vi "FIR Windowed Filter Design - DFD.vi"() -> ()   [LabVIEW 2023]
doc: "Demonstrates how to design an FIR windowed filter using VIs in the LabVIEW Digital Filter Design Toolkit. \n\nAs you change the Filter Type, experiment with the parameters for that filter type and observe their effect on the magnitude and phase responses."
uses:
  <vilib>/addons/Digital Filter Design/_Objects.llb/DFD Phase Setting.ctl
  <vilib>/addons/Digital Filter Design/Analysis.llb/DFD Plot Freq Response (Linear-Spaced).vi
  <vilib>/addons/Digital Filter Design/NI_DigFilterLicensed.lvlib
panel:
  out "?":string="dB"
  in  "window":i32(ring)=1 items=["None", "Hanning", "Hamming", "Triangular", "Blackman", "Exact Blackman", "Blackman-Harris", "Kaiser-Bessel", "Flat Top"]
  in  "high cutoff freq: fh":dbl=350.0 format="%0.2f"
  in  "low cutoff freq: fl":dbl=150.0 format="%0.2f"
  in  "sampling frequency: fs":dbl=1000.0 format="%0.2f"
  in  "Display":bool=TRUE
  in  "stop":bool
  in  "Filter Type":T1(ring)=enum."Bandpass"
  in  "taps":i32=33
  out "Phase Response":cluster{"f0":dbl, "df":dbl, "values":dbl[]}[](graph)
  out "Magnitude Response":cluster{"f0":dbl, "df":dbl, "values":dbl[]}[](graph)
  # "Select Help»Show Context Help and move the cursor over the VI icon for more information."
  # "Hz"
  # "radians"
  # "Hz"
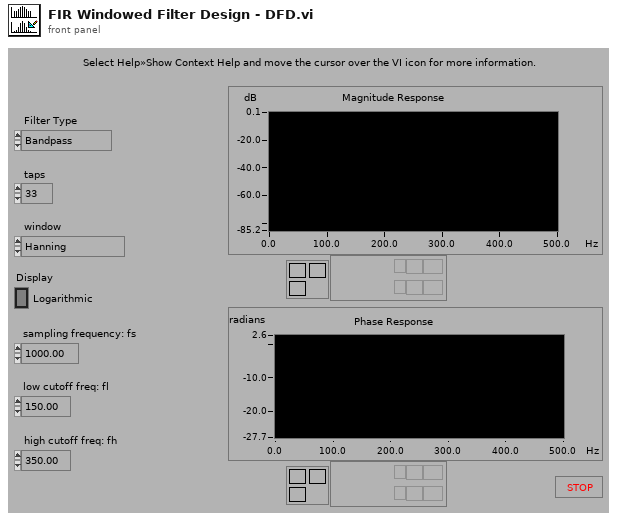
[diagram p1: front panel]
types:
  T1 = enum16{"Lowpass", "Highpass", "Bandpass", "Bandstop"}
  T2 = typedef "NI_DigFilterLicensed.lvlib/DFD Phase Setting.ctl" = cluster{"unwrap? (F)":bool, "degree? (F)":bool}
  T3 = typedef "NI_DigFilterLicensed.lvlib/DFD Filter Obj.ctl" = cluster{"mSRate_Fs":dbl, "mSRate_Version":string, "mSRate_Comments":string, "mSRate_OrgCoef":T4, "mSRate_CurCoef":T4, "mSRate_Quantized?":bool, "mSRate_QCoef":T4, "mSRate_QSettings":T6[], "mSRate_Order":i32, "mSRate_Scaling":cluster{"mSRate_ScaleByPowerOf2?":bool, "mSRate_ScaleType":T8}}
  T4 = typedef "NI_DigFilterLicensed.lvlib/DFD Filter Coef.ctl" = cluster{"type":T5, "gain":dbl, "coef a (k)":dbl[], "coef b (v)":dbl[]}
  T5 = typedef "NI_DigFilterLicensed.lvlib/DFD Filter Structure Type Selector.ctl" = enum16{"Undefined", "FIR Direct Form", "FIR Direct Form Transposed", "FIR Symmetric", "FIR Antisymmetric", "IIR Direct Form I", "IIR Direct Form I Transposed", "IIR Direct Form II", "IIR Direct Form II Transposed", "IIR Cascaded Second Order Sections Form I", "IIR Cascaded Second Order Sections Form I Transposed", "IIR Cascaded Second Order Sections Form II", "IIR Cascaded Second Order Sections Form II Transposed", "Lattice Allpass (basic sections)", "Lattice Allpass (one multiplier sections)", "Lattice Allpass (normalized sections)", "Lattice AR (basic sections)", "Lattice AR (one multiplier sections)", "Lattice AR (normalized sections)", "Lattice MA (minimum phase)", "Lattice MA (maximum phase)", "Lattice ARMA (basic sections)", "Lattice ARMA (one multiplier sections)", "Lattice ARMA (normalized sections)"}
  T6 = typedef "NI_DigFilterLicensed.lvlib/dfd_Internal Quantization Settings.ctl" = cluster{"source":T7, "wl":i16, "iwl":i16, "overflow mode":enum16{"Saturation", "Wrap"}, "rounding mode":enum16{"Nearest", "Truncation"}, "signed?":bool}
  T7 = typedef "NI_DigFilterLicensed.lvlib/dfd_Internal Quantization Srcs.ctl" = u16
  T8 = typedef "NI_DigFilterLicensed.lvlib/DFD Coef Norm Type.ctl" = enum16{"No Norm", "Time Domain 1-Norm", "Time Domain 2-Norm", "Time Domain Inf-Norm"}
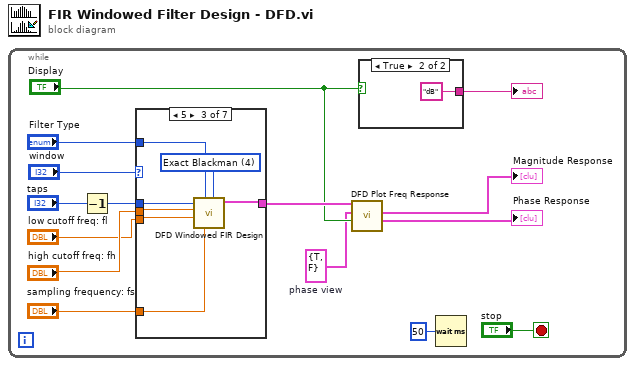
[diagram p0: block diagram]
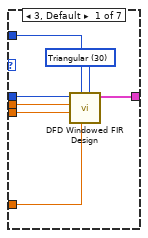
[diagram p2: hidden frame]
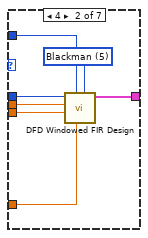
[diagram p3: hidden frame]
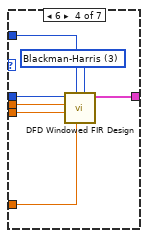
[diagram p4: hidden frame]
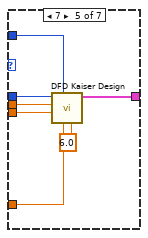
[diagram p5: hidden frame]
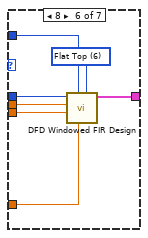
[diagram p6: hidden frame]
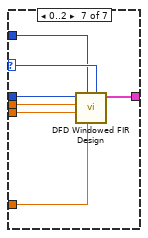
[diagram p7: hidden frame]
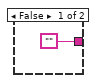
[diagram p8: hidden frame]
diagram:
  n1 = while {
    stop <- "stop" stop-if-true
    w1 = T2 {"unwrap? (F)"=TRUE, "degree? (F)"=FALSE}  # phase view
    n2 = Decrement(x="taps") -> (x-1=w11:i32)
    n3 = case shown="5" "window" {
      selector: "window" -> [_ _ _ _ _ _ w63]
      tunnel: w11 -> [w20 w28 w35 w42 w50 w56 w64]
      tunnel: "Filter Type" -> [w21 w25 w32 w37 w45 w51 w62]
      tunnel: "high cutoff freq: fh" -> [w19 w27 w34 w41 w49 w55 w61]
      tunnel: "low cutoff freq: fl" -> [w18 w26 w33 w40 w48 w54 w60]
      tunnel: "sampling frequency: fs" -> [w17 w23 w30 w38 w47 w52 w59]
      tunnel: [w16 w24 w31 w39 w46 w53 w58] -> w5
      frame 3, Default {
        w22 = u16 30 items=["None"=0, "Hanning"=1, "Hamming"=2, "Blackman-Harris"=3, "Exact Blackman"=4, "Blackman"=5, "Flat Top"=6, "4 Term B-Harris"=7, "7 Term B-Harris"=8, "Low Sidelobe"=9, "Triangular"=30] ("window")
        n4 = call <vilib>:"DFD Windowed FIR Design.vi"("window"=w22, "fs [Hz]"=w17, "filter type"=w21, "low cutoff freq [Hz]"=w18, "high cutoff freq [Hz]"=w19, "order"=w20) -> ("filter out"=w16:T3)  [unwired: 2 in, 3 out]
      }
      frame 4 {
        w29 = u16 5 items=["None"=0, "Hanning"=1, "Hamming"=2, "Blackman-Harris"=3, "Exact Blackman"=4, "Blackman"=5, "Flat Top"=6, "4 Term B-Harris"=7, "7 Term B-Harris"=8, "Low Sidelobe"=9, "Triangular"=30] ("window")
        n5 = call <vilib>:"DFD Windowed FIR Design.vi"("window"=w29, "fs [Hz]"=w23, "filter type"=w25, "low cutoff freq [Hz]"=w26, "high cutoff freq [Hz]"=w27, "order"=w28) -> ("filter out"=w24:T3)  [unwired: 2 in, 3 out]
      }
      frame 5 {
        w36 = u16 4 items=["None"=0, "Hanning"=1, "Hamming"=2, "Blackman-Harris"=3, "Exact Blackman"=4, "Blackman"=5, "Flat Top"=6, "4 Term B-Harris"=7, "7 Term B-Harris"=8, "Low Sidelobe"=9, "Triangular"=30] ("window")
        n6 = call <vilib>:"DFD Windowed FIR Design.vi"("window"=w36, "fs [Hz]"=w30, "filter type"=w32, "low cutoff freq [Hz]"=w33, "high cutoff freq [Hz]"=w34, "order"=w35) -> ("filter out"=w31:T3)  [unwired: 2 in, 3 out]
      }
      frame 6 {
        w43 = u16 3 items=["None"=0, "Hanning"=1, "Hamming"=2, "Blackman-Harris"=3, "Exact Blackman"=4, "Blackman"=5, "Flat Top"=6, "4 Term B-Harris"=7, "7 Term B-Harris"=8, "Low Sidelobe"=9, "Triangular"=30] ("window")
        n7 = call <vilib>:"DFD Windowed FIR Design.vi"("window"=w43, "fs [Hz]"=w38, "filter type"=w37, "low cutoff freq [Hz]"=w40, "high cutoff freq [Hz]"=w41, "order"=w42) -> ("filter out"=w39:T3)  [unwired: 2 in, 3 out]
      }
      frame 7 {
        n8 = call <vilib>:"DFD Kaiser Design.vi"("beta"=6.0, "fs [Hz]"=w47, "filter type"=w45, "low cutoff freq [Hz]"=w48, "high cutoff freq [Hz]"=w49, "order"=w50) -> ("filter out"=w46:T3)  [unwired: 1 in, 4 out]
      }
      frame 8 {
        w57 = u16 6 items=["None"=0, "Hanning"=1, "Hamming"=2, "Blackman-Harris"=3, "Exact Blackman"=4, "Blackman"=5, "Flat Top"=6, "4 Term B-Harris"=7, "7 Term B-Harris"=8, "Low Sidelobe"=9, "Triangular"=30] ("window")
        n9 = call <vilib>:"DFD Windowed FIR Design.vi"("window"=w57, "fs [Hz]"=w52, "filter type"=w51, "low cutoff freq [Hz]"=w54, "high cutoff freq [Hz]"=w55, "order"=w56) -> ("filter out"=w53:T3)  [unwired: 2 in, 3 out]
      }
      frame 0..2 {
        n10 = call <vilib>:"DFD Windowed FIR Design.vi"("window"=w63, "fs [Hz]"=w59, "filter type"=w62, "low cutoff freq [Hz]"=w60, "high cutoff freq [Hz]"=w61, "order"=w64) -> ("filter out"=w58:T3)  [unwired: 2 in, 3 out]
      }
    }
    n11 = call-poly <vilib>:"DFD Plot Freq Response.vi"("dB on? (T)"="Display", "phase view"=w1, "filter in"=w5) -> ("phase response"=→"Phase Response":cluster{"f0":dbl, "df":dbl, "values":dbl[]}[], "magnitude response"=→"Magnitude Response":cluster{"f0":dbl, "df":dbl, "values":dbl[]}[])  [unwired: 5 in, 2 out]
    n12 = case shown="True" "Display" {
      tunnel: ["" "dB"] -> w15
      frame False {
      }
      frame True {
      }
    }
    "?" <- w15
    n13 = Wait (ms)(milliseconds to wait=u32 50) -> ()  [unwired: 1 out]
  }
